vi "SVT Convert FFT Spectrum to CPB Spectrum (1 Ch).vi"(0 "spectrum":cluster{"x0":dbl, "dx":dbl, "magnitude":dbl[]} {"magnitude" format="%.2f"; "dx" format="%.2f"; "x0" format="%.2f"}, 1 "frequency range [Hz]":cluster{"start":dbl, "stop":dbl}={"start"=20.0, "stop"=20000.0} {"stop" format="%.2f"; "start" format="%.2f"}, 2 "bandwidth":T1(ring)=enum."1/3 octave", 4 "spectrum info":T7={"channel name"="", "description"="", "x-axis units"=0, "spectral info"={"spectrum type"=enum."Power [Magnitude^2]", "linear/dB"=enum."linear", "window"=0, "window size"=0, "FFT size"=0}, "engineering units"=0, "custom label"="", "dB reference [EU]"=0.0, "peak units"=enum."rms", "weighting filter"=0, "spectral density?"=FALSE, "unit label"="", "spectrum skewed?"=FALSE, "complimentary spectrum units"=enum."none"} {"x-axis units" items=["Time (s)"=0, "Frequency-CB (Hz)"=1, "Frequency-CPB (Hz)"=1248, "Frequency-Arbitrary (Hz)"=2357, "Quefrency (s)"=2, "Revolutions (rev)"=3, "Order"=4, "Speed (RPM)"=11, "Speed (rad/s)"=21, "Index"=65535]; "weighting filter" items=["Linear", "A-weighting", "B-weighting", "C-weighting", "ITU-R 468-4", "Dolby", "CCITT", "C-message", "Wb", "Wc", "Wd", "We", "Wf", "Wh", "Wj", "Wk", "Wm", "AES17 20 kHz lowpass", "AES17 40 kHz lowpass", "AES17 20 kHz highpass", "AES17 40 kHz highpass"]; "dB reference [EU]" format="%.2f"; "engineering units" items=["custom..."=0, "V"=1, "A"=21, "C"=30, "pC"=31, "s"=32, "-"=29, "Pa"=2, "N"=20, "g"=3, "m/s^2"=4, "m/s"=5, "m"=6, "mm/s"=12, "mm"=13, "micron/s"=14, "micron"=15, "in/s^2"=7, "in/s"=8, "in"=9, "mil/s"=10, "mil"=11, "rad/s^2"=16, "rad/s"=17, "rad"=18, "deg/s^2"=26, "deg/s"=27, "deg"=28, "RPM"=22, "cycle/s^2"=23, "Hz"=24, "cycle"=25, "strain"=19]; "spectral info"."window" items=["None "=0, "Hanning"=1, "Hamming"=2, "Blackman-Harris"=3, "Exact Blackman"=4, "Blackman"=5, "Flat Top"=6, "4 Term B-Harris "=7, "7 Term B-Harris"=8, "Low Sidelobe"=9, "Force - Exponential"=10, "Gaussian"=62]}, 5 "error in (no error)":errorcluster) -> (14 "octave spectrum":T6 {"band power" format="%.2f"; "nominal frequencies [Hz]" format="%.2f"}, 15 "unit label":string, 16 "total band power":dbl=nan format="%.2f", 18 "octave info":T2={"standard"=enum."ANSI S1.11", "bandwidth"=enum."1 octave", "low band"=0, "high band"=0, "weighting filter"=0, "dB reference"=0.0, "dB On"=FALSE, "unit label"="", "channel name"="", "description"="", "engineering units"=1, "custom label"="", "spectrum type"=enum."magnitude", "spectral density"=FALSE, "filters settled"=FALSE} {"engineering units" items=["custom..."=0, "V"=1, "A"=21, "C"=30, "pC"=31, "s"=32, "-"=29, "Pa"=2, "N"=20, "g"=3, "m/s^2"=4, "m/s"=5, "m"=6, "mm/s"=12, "mm"=13, "micron/s"=14, "micron"=15, "in/s^2"=7, "in/s"=8, "in"=9, "mil/s"=10, "mil"=11, "rad/s^2"=16, "rad/s"=17, "rad"=18, "deg/s^2"=26, "deg/s"=27, "deg"=28, "RPM"=22, "cycle/s^2"=23, "Hz"=24, "cycle"=25, "strain"=19]; "dB reference" format="%.2e"; "weighting filter" items=["Linear", "A-weighting", "B-weighting", "C-weighting", "ITU-R 468-4", "Dolby", "CCITT", "C-message", "Wb", "Wc", "Wd", "We", "Wf", "Wh", "Wj", "Wk", "Wm", "AES17 20 kHz lowpass", "AES17 40 kHz lowpass", "AES17 20 kHz highpass", "AES17 40 kHz highpass"]}, 19 "error out":errorcluster)   [LabVIEW 2017, in "SoundVib_Octave_2014 standard.lvlib"]
doc: "Computes the aggregate power in the <B>range</B>. The SVL Power in Band VI operates on Power, PSD, COP, and FFT [Mag] spectra. You can use this polymorphic VI to analyze a single spectrum or N spectra. The data type you wire to the <B>spectrum</B> input determines the polymorphic instance to use."
uses:
  <vilib>/addons/Sound and Vibration/svt_Octave/SoundVib_Octave_2014 standard.lvlib
  <vilib>/addons/_NISVFA/_Shared subVIs/Controls/svc_Spectrum Info.ctl
  <vilib>/addons/_NISVFA/_Shared subVIs/Controls/svc_X-Axis Units.ctl
  <vilib>/addons/_NISVFA/_Shared subVIs/Controls/svc_Spectrum Type.ctl
  <vilib>/addons/_NISVFA/_Shared subVIs/Controls/svc_Engineering Units Text Ring.ctl
  <vilib>/addons/_NISVFA/_Shared subVIs/Controls/svc_Weighting Filter Text Ring.ctl
  <vilib>/addons/_NISVFA/_Shared subVIs/Controls/svc_Complimentary Spectrum Units.ctl
  <vilib>/addons/_NISVFA/_Shared subVIs/Controls/svc_Octave Info.ctl
  <vilib>/addons/_NISVFA/_Shared subVIs/Controls/svc_Octave Standard.ctl
  <vilib>/addons/_NISVFA/_Spectrum Processing/SVFA Unit Conversion (1 Ch).vi
  <vilib>/addons/_NISVFA/_Shared subVIs/Common/svc_Spectrum Units.vi
  <vilib>/addons/_NISVFA/_Spectrum Processing/subVIs/svfa_Conversion Utility (spectrum info).vi
  <vilib>/addons/_NISVFA/_Spectrum Processing/subVIs/svfa_Peak to RMS to Peak2Peak.vi
  <vilib>/addons/_NISVFA/_Spectrum Processing/subVIs/svfa_Mag to Mag2.vi
  <vilib>/addons/_NISVFA/_Spectrum Processing/subVIs/svfa_Linear to dB.vi
  <vilib>/addons/_NISVFA/_Spectrum Processing/subVIs/svfa_dBrefA to dBrefB.vi
  <vilib>/addons/_NISVFA/_Spectrum Processing/subVIs/svfa_Spectrum to Spectral Density.vi
  <vilib>/addons/_NISVFA/_Shared subVIs/Common/svc_Get Weighting Enum and Labels.vi
  <vilib>/addons/_NISVFA/_Shared subVIs/Common/svc_Unit Label Lexical Class.vi
  <vilib>/addons/_NISVFA/_Shared subVIs/Common/svc_Engineering Units to Unit Label.vi
  <vilib>/addons/_NISVFA/_Shared subVIs/Common/svc_Format Value (DBL).vi
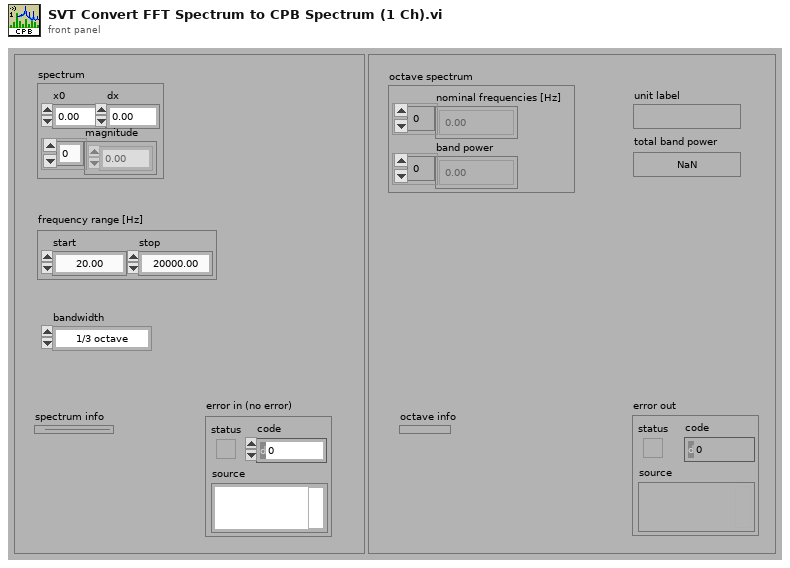
[diagram p1: front panel]
types:
  T1 = enum16{"1 octave", "1/3 octave", "1/6 octave", "1/12 octave", "1/24 octave", "1/48 octave", "1/96 octave"}
  T2 = typedef "svc_Octave Info.ctl" = cluster{"standard":T3, "bandwidth":enum16{"1 octave", "1/3 octave", "1/6 octave", "1/12 octave", "1/24 octave"}, "low band":i32, "high band":i32, "weighting filter":T4, "dB reference":dbl, "dB On":bool, "unit label":string, "channel name":string, "description":string, "engineering units":T5, "custom label":string, "spectrum type":enum16{"power", "magnitude"}, "spectral density":bool, "filters settled":bool}
  T3 = typedef "svc_Octave Standard.ctl" = enum16{"ANSI S1.11", "IEC 61260"}
  T4 = typedef "svc_Weighting Filter Text Ring.ctl" = u16
  T5 = typedef "svc_Engineering Units Text Ring.ctl" = u16
  T6 = cluster{"nominal frequencies [Hz]":dbl[], "band power":dbl[]}
  T7 = typedef "svc_Spectrum Info.ctl" = cluster{"channel name":string, "description":string, "x-axis units":T8, "spectral info":cluster{"spectrum type":T9, "linear/dB":enum16{"linear", "dB"}, "window":u16, "window size":i32, "FFT size":i32}, "engineering units":T5, "custom label":string, "dB reference [EU]":dbl, "peak units":enum16{"rms", "peak", "peak-peak"}, "weighting filter":T4, "spectral density?":bool, "unit label":string, "spectrum skewed?":bool, "complimentary spectrum units":T10}
  T8 = typedef "svc_X-Axis Units.ctl" = u16
  T9 = typedef "svc_Spectrum Type.ctl" = enum16{"FFT Spectrum [complex]", "Amplitude [Magnitude]", "Power [Magnitude^2]", "Cross Spectrum [complex]", "Frequency Response [Complex]"}
  T10 = typedef "svc_Complimentary Spectrum Units.ctl" = enum16{"none", "radians", "degrees", "cycles", "imaginary"}
  T11 = cluster{"linear/dB":enum16{"no change", "linear", "dB"}, "dB reference (0: no change)":dbl, "power/magnitude":enum16{"no change", "power", "magnitude"}, "view":enum16{"no change", "rms", "peak", "peak-peak"}}
  T12 = enum16{"no change", "spectrum", "spectral density"}
  T13 = cluster{"f low":dbl, "f high":dbl, "midband":dbl}[]
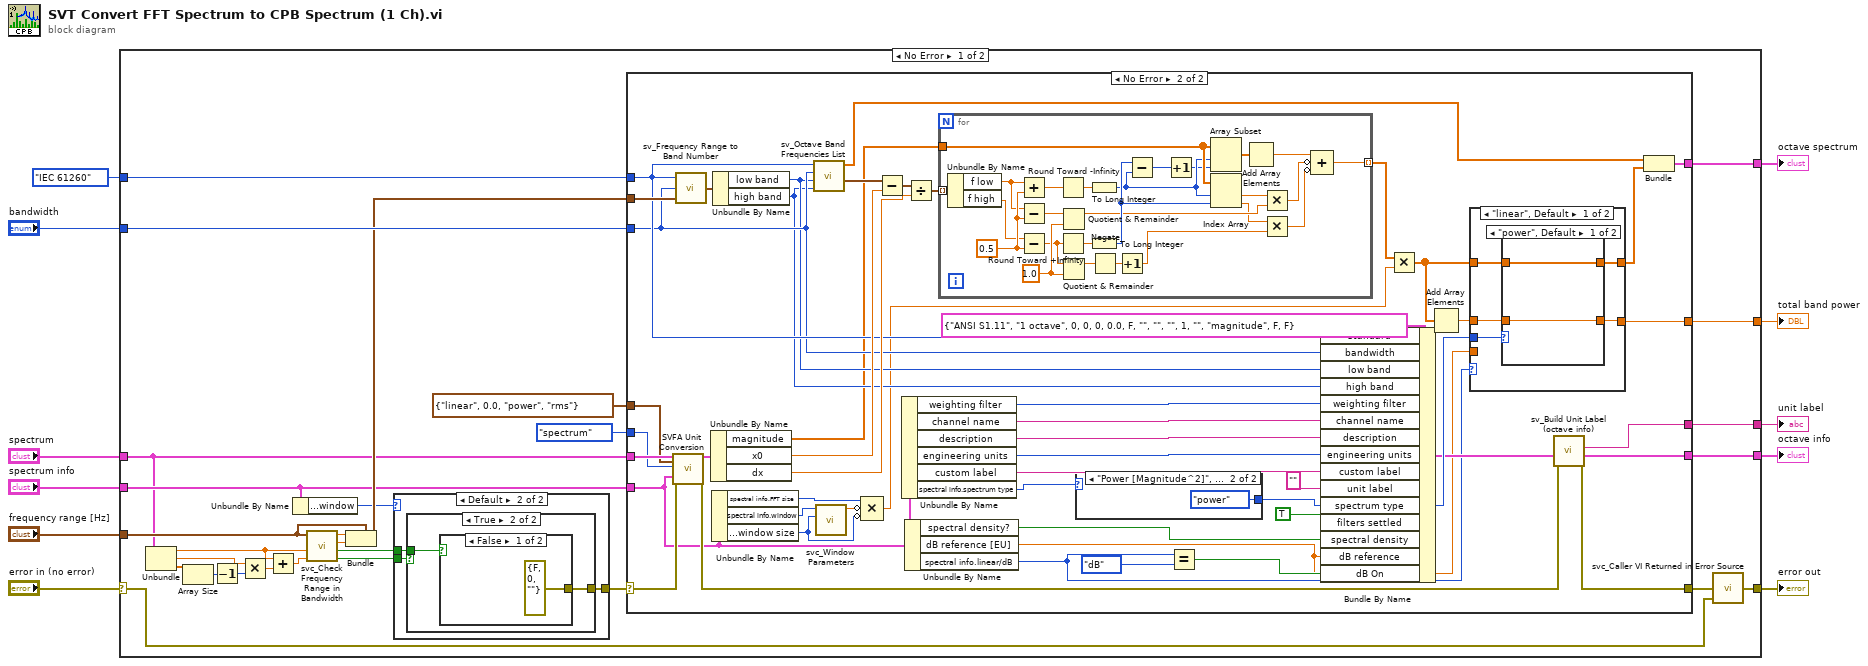
[diagram p0: block diagram]
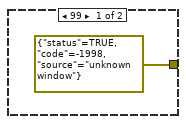
[diagram p2: hidden frame]
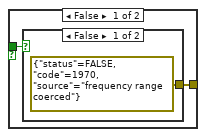
[diagram p3: hidden frame]
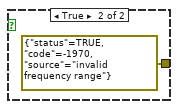
[diagram p4: hidden frame]
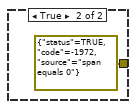
[diagram p5: hidden frame]
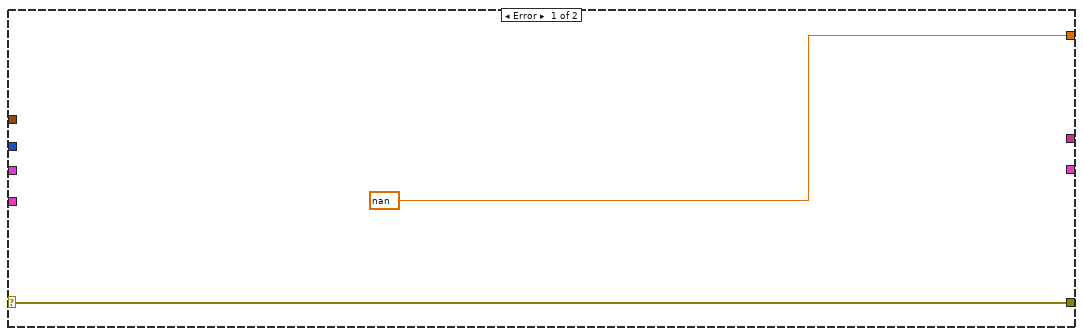
[diagram p6: hidden frame]
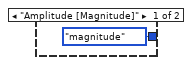
[diagram p7: hidden frame]
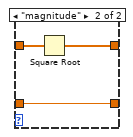
[diagram p8: hidden frame]
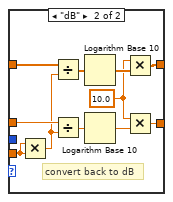
[diagram p9: hidden frame]
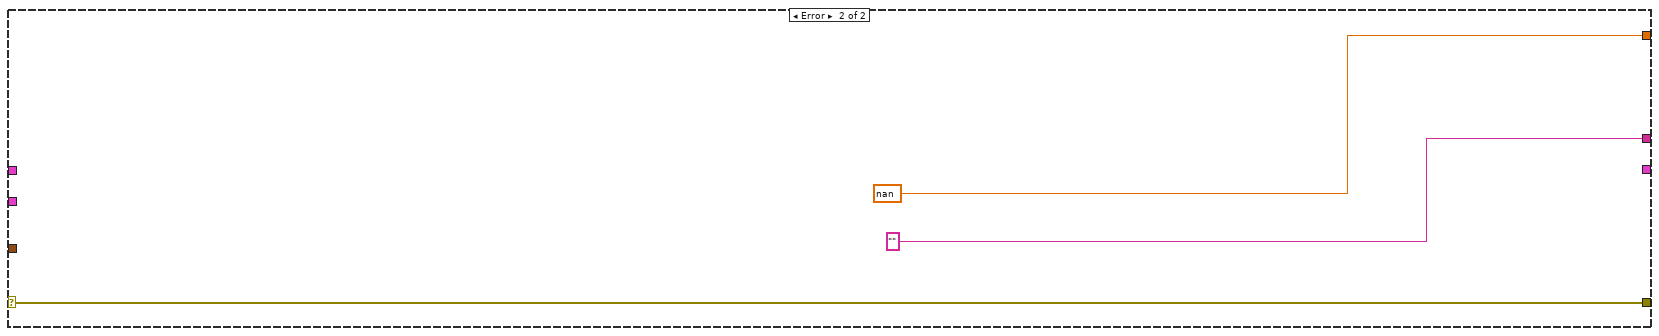
[diagram p10: hidden frame]
diagram:
  n1 = case shown="No Error" "error in (no error)" {
    selector: "error in (no error)" -> [w21 w155]
    tunnel: "spectrum" -> [w17 _]
    tunnel: [w36 nan ("power in band")] -> w10
    tunnel: [w39 w155] -> w9
    tunnel: "frequency range [Hz]" -> [w24 _]
    tunnel: "spectrum info" -> [w18 _]
    tunnel: [w15 "" ("unit label")] -> w7
    tunnel: "bandwidth" -> [w38 _]
    tunnel: svc_Octave_Standard."IEC 61260" ("standard") -> [w37 _]
    tunnel: [w16 _] -> w2
    tunnel: [w14 _] -> w1
    frame No Error {
      n2 = Unbundle(w17) -> ("x0"=w29:dbl, "dx"=w30:dbl, "magnitude"=w34:dbl[])
      n3 = Array Size(array=w34) -> (size(s)=w32:i32)
      n4 = Decrement(x=w32) -> (x-1=w31:i32)
      n5 = Multiply(x=w30, y=w31) -> (x*y=w33:dbl)
      n6 = Add(x=w29, y=w33) -> (x+y=w28:dbl)
      n7 = Unbundle By Name(w18) -> ("spectral info.window"=w19:u16)
      n8 = call <vilib>:"svc_Check Frequency Range in Bandwidth.vi"("fmax"=w28, "fmin"=w29, "frequency range"=w24) -> ("start and stop in range"=w23:bool, "zero span"=w22:bool, "stop frequency"=w25:dbl, "start frequency"=w26:dbl)  [unwired: 5 in]
      n9 = Bundle(cluster=w24, "start"=w26, "stop"=w25) -> (w27:cluster{"start":dbl, "stop":dbl})
      n10 = case shown="Default" w19 {
        tunnel: w23 -> [_ w43]
        tunnel: w22 -> [_ w42]
        tunnel: [errorcluster {"status"=TRUE, "code"=-1998, "source"="unknown window"} ("error out") w41] -> w20
        frame 99 {
        }
        frame Default {
          n11 = case shown="True" w43 {
            tunnel: [w45 w48] -> w41
            tunnel: w42 -> [w44 w49]
            frame False {
              n12 = case shown="False" w44 {
                tunnel: [errorcluster {"status"=FALSE, "code"=1970, "source"="frequency range coerced"} ("error in (no error)") errorcluster {"status"=TRUE, "code"=-1970, "source"="invalid frequency range"} ("error in (no error)")] -> w45
                frame False {
                }
                frame True {
                }
              }
            }
            frame True {
              n13 = case shown="False" w49 {
                tunnel: [errorcluster {"status"=FALSE, "code"=0, "source"=""} ("error out") errorcluster {"status"=TRUE, "code"=-1972, "source"="span equals 0"} ("error out")] -> w48
                frame False {
                }
                frame True {
                }
              }
            }
          }
        }
      }
      n14 = case shown="No Error" w20 {
        selector: w20 -> [w53 w82]
        tunnel: w17 -> [_ w100]
        tunnel: w18 -> [_ w72]
        tunnel: w27 -> [_ w99]
        tunnel: w38 -> [_ w90]
        tunnel: w37 -> [_ w91]
        tunnel: [nan w93] -> w36
        tunnel: [w53 w77] -> w35
        tunnel: [_ w81] -> w16
        tunnel: [_ w76] -> w15
        tunnel: [_ w79] -> w14
        tunnel: T11 {"linear/dB"=enum."linear", "dB reference (0: no change)"=0.0, "power/magnitude"=enum."power", "view"=enum."rms"} ("desired scaling") -> [_ w75]
        tunnel: T12."spectrum" ("spectral density desired") -> [_ w74]
        frame Error {
        }
        frame No Error {
          n15 = call-poly <vilib>:"SVFA Unit Conversion.vi"("spectrum"=w100, "desired scaling"=w75, "spectral density desired"=w74, "spectrum info in"=w72, "error in (no error)"=w82) -> ("converted spectrum"=w103:cluster{"x0":dbl, "dx":dbl, "magnitude":dbl[]}, "error out"=w78:errorcluster)  [unwired: 11 in, 2 out]
          n16 = call <vilib>:"sv_Frequency Range to Band Number.vi"("frequency range [Hz]"=w99, "bandwidth"=w90, "standard"=w91) -> ("band number"=w101:cluster{"low band":i32, "high band":i32})
          n17 = Unbundle By Name(w103) -> ("magnitude"=w55:dbl[], "x0"=w98:dbl, "dx"=w96:dbl)
          n18 = Unbundle By Name(w72) -> ("spectral info.FFT size"=w61:i32, "spectral info.window"=w62:u16, "spectral info.window size"=w59:i32)
          n19 = Unbundle By Name(w101) -> ("low band"=w89:i32, "high band"=w88:i32)
          n20 = call <vilib>:"sv_Octave Band Frequencies List.vi"("high band selector"=w88, "low band selector"=w89, "bandwidth"=w90, "standard"=w91) -> ("bandedge frequencies [Hz]"=w97:T13, "nominal frequencies [Hz]"=w73:dbl[])  [unwired: 4 in, 2 out]
          n21 = call <vilib>:"svc_Window Parameters.vi"("window size"=w59, "window"=w62) -> ("ENBW"=w60:dbl)  [unwired: 6 in, 3 out]
          n22 = Compound Arithmetic op=MULTIPLY(w61, invert w60, invert w59) -> (w58:dbl)
          n23 = Subtract(x=w97, y=w98) -> (x-y=w102:T13)
          n24 = Unbundle By Name(w72) -> ("weighting filter"=w66:T4, "channel name"=w67:string, "description"=w68:string, "engineering units"=w69:T5, "custom label"=w70:string, "spectral info.spectrum type"=w71:T9)
          n25 = Unbundle By Name(w72) -> ("spectral density?"=w65:bool, "dB reference [EU]"=w64:dbl, "spectral info.linear/dB"=w63:enum16{"linear", "dB"})
          n26 = Divide(x=w102, y=w96) -> (x/y=w56:T13)
          n27 = for {
            tunnel: w56 -> [w129] mode=indexing
            tunnel: w55 -> [w128]
            tunnel: [w127] -> w54 mode=indexing
            w118 = 0.5 ("x")
            w122 = 1.0 ("y")
            n28 = Unbundle By Name(w129) -> ("f low"=w111:dbl, "f high"=w112:dbl)
            n29 = Add(x=w111, y=w118) -> (x+y=w125:dbl)
            n30 = Subtract(x=w111, y=w118) -> (x-y=w119:dbl)
            n31 = Subtract(x=w112, y=w118) -> (x-y=w115:dbl)
            n32 = Round Toward -Infinity(1:w125) -> (0:w124:dbl)
            n33 = Round Toward +Infinity(x=w115) -> (ceil(x): smallest int >= x=w126:dbl)
            n34 = Quotient & Remainder(x=w119, y=w122) -> (x-y*floor(x/y)=w114:dbl)  [unwired: 1 out]
            n35 = Quotient & Remainder(x=w115, y=w122) -> (x-y*floor(x/y)=w117:dbl)  [unwired: 1 out]
            n36 = To Long Integer(number=w124) -> (32bit integer=w121:i32)
            n37 = To Long Integer(number=w126) -> (32bit integer=w123:i32)
            n38 = Negate(x=w117) -> (-x=w116:dbl)
            n39 = Increment(x=w116) -> (x+1=w113:dbl)
            n40 = Subtract(x=w123, y=w121) -> (x-y=w120:i32)
            n41 = Increment(x=w120) -> (x+1=w106:i32)
            n42 = Array Subset(array=w128, index=w121, length=w106) -> (w107:dbl[])
            n43 = Index Array(array=w128, index #1=w121, index #2=w123) -> (element #1=w105:dbl, element #2=w104:dbl)
            n44 = Add Array Elements(numeric array=w107) -> (sum=w110:dbl)
            n45 = Multiply(x=w105, y=w114) -> (x*y=w109:dbl)
            n46 = Multiply(x=w104, y=w113) -> (x*y=w108:dbl)
            n47 = Compound Arithmetic op=ADD(w110, invert w109, invert w108) -> (w127:dbl)
          }
          n48 = case shown="\"Power [Magnitude^2]\", Default" w71 {
            tunnel: [enum16{"power", "magnitude"}."magnitude" ("spectrum type") enum16{"power", "magnitude"}."power" ("spectrum type")] -> w83
            frame "Amplitude [Magnitude]" {
            }
            frame "Power [Magnitude^2]", Default {
            }
          }
          n49 = Equal?(x=w63, y=enum16{"linear", "dB"}."dB" ("x")) -> (x = y?=w84:bool)
          n50 = Bundle By Name(cluster=T2 {"standard"=enum."ANSI S1.11", "bandwidth"=enum."1 octave", "low band"=0, "high band"=0, "weighting filter"=0, "dB reference"=0.0, "dB On"=FALSE, "unit label"="", "channel name"="", "description"="", "engineering units"=1, "custom label"="", "spectrum type"=enum."magnitude", "spectral density"=FALSE, "filters settled"=FALSE} ("octave info"), "standard"=w91, "bandwidth"=w90, "low band"=w89, "high band"=w88, "weighting filter"=w66, "channel name"=w67, "description"=w68, "engineering units"=w69, "custom label"=w70, "unit label"="", "spectrum type"=w83, "filters settled"=TRUE, "spectral density"=w65, "dB reference"=w64, "dB On"=w84) -> (w80:T2)
          n51 = Multiply(x=w54, y=w58) -> (x*y=w57:dbl[])
          n52 = Add Array Elements(numeric array=w57) -> (sum=w94:dbl)
          n53 = case shown="\"linear\", Default" w63 {
            tunnel: [w133 w152] -> w95
            tunnel: w57 -> [w134 w150]
            tunnel: w64 -> [_ w148]
            tunnel: w94 -> [w135 w145]
            tunnel: [w132 w143] -> w93
            tunnel: w83 -> [w136 _]
            frame "linear", Default {
              n54 = case shown="\"power\", Default" w136 {
                tunnel: w135 -> [w137 w140]
                tunnel: w134 -> [w138 w141]
                tunnel: [w138 w139] -> w133
                tunnel: [w137 w140] -> w132
                frame "power", Default {
                }
                frame "magnitude" {
                  n55 = Square Root(x=w141) -> (sqrt(x)=w139:dbl[])
                }
              }
            }
            frame "dB" {
              w142 = 10.0 ("Numeric")
              # "convert back to dB"
              n56 = Multiply(x=w148, y=w148) -> (x*y=w144:dbl)
              n57 = Divide(x=w150, y=w144) -> (x/y=w149:dbl[])
              n58 = Divide(x=w145, y=w144) -> (x/y=w147:dbl)
              n59 = Logarithm Base 10(1:w149) -> (0:w151:dbl[])
              n60 = Logarithm Base 10(1:w147) -> (0:w146:dbl)
              n61 = Multiply(x=w142, y=w151) -> (x*y=w152:dbl[])
              n62 = Multiply(x=w142, y=w146) -> (x*y=w143:dbl)
            }
          }
          n63 = call <vilib>:"sv_Build Unit Label (octave info).vi"("error in (no error)"=w78, "octave info"=w80) -> ("error out"=w77:errorcluster, "octave info out"=w79:T2, "unit label"=w76:string)  [unwired: 7 in]
          n64 = Bundle("nominal frequencies [Hz]"=w73, w95) -> (w81:cluster{"nominal frequencies [Hz]":dbl[], dbl[]})  [unwired: 1 in]
        }
      }
      n65 = call <vilib>:"svc_Caller VI Returned in Error Source.vi"("warning input to caller"=w21, "error in (no error)"=w35) -> ("error out"=w39:errorcluster)  [unwired: 3 in]
    }
    frame Error {
    }
  }
  "error out" <- w9
  "total band power" <- w10
  "unit label" <- w7
  "octave info" <- w1
  "octave spectrum" <- w2
